vi "Calcul Tarifs Bourse.vi"(11 "Provider":T1) -> (2 "Graphe":dbl[](graph))   [LabVIEW 2012]
uses:
  PortFolio-Provider.ctl
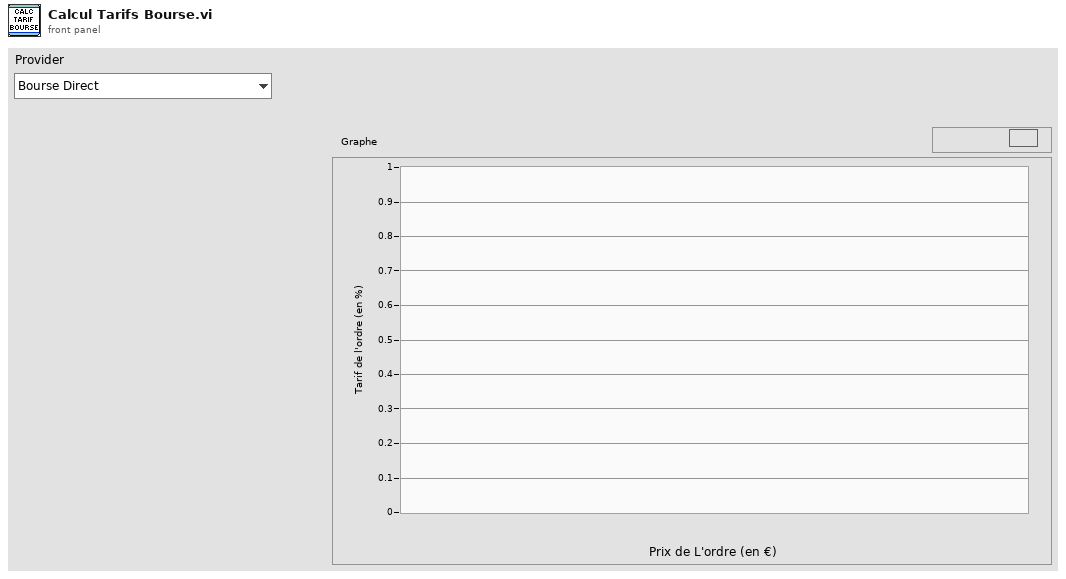
[diagram p1: front panel]
types:
  T1 = typedef "PortFolio-Provider.ctl" = enum16{"Bourse Direct", "Binck classique", "Boursorama Découverte", "Boursorama Classique", "Boursorama Trader", "Boursorama Ultimate Trader", "IG Actions Euro"}
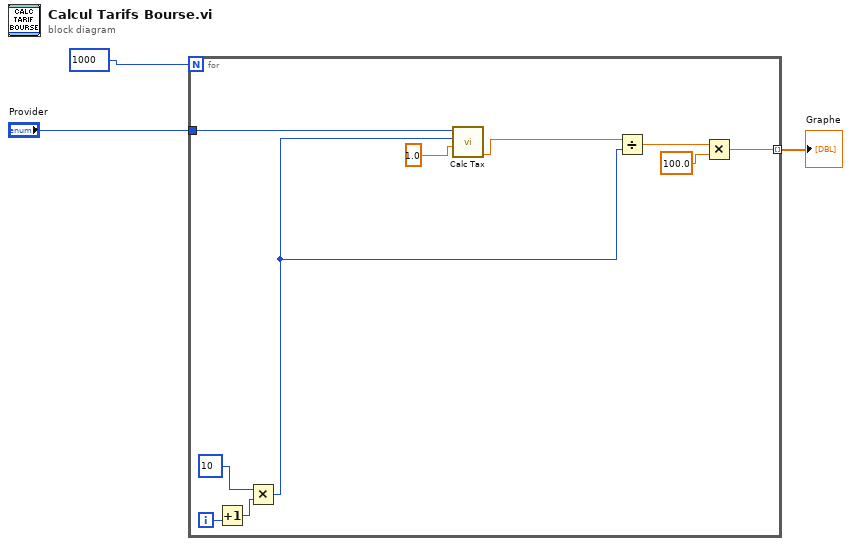
[diagram p0: block diagram]
diagram:
  n1 = for {
    N: 1000 -> [_]
    tunnel: "Provider" -> [w13]
    tunnel: [w5] -> w1 mode=indexing
    i -> [w9]
    n2 = Increment(x=w9) -> (x+1=w8:i32)
    n3 = Multiply(x=10, y=w8) -> (x*y=w10:i32)
    n4 = call "Calc Tax.vi"("Price"=1.0, "Qty"=w10, "Provider"=w13) -> ("Cout Plateforme"=w4:dbl)  [unwired: 7 in, 1 out]
    n5 = Divide(x=w4, y=w10) -> (x/y=w7:dbl)
    n6 = Multiply(x=w7, y=100.0) -> (x*y=w5:dbl)
  }
  "Graphe" <- w1
